vi "Prepare_ Trajectory.vi"(0 "reference in":refnum<class "Manipulator.lvclass">, 11 "error in (no error)":errorcluster) -> (4 "reference out":refnum<class "Manipulator.lvclass">, 6 "X":dbl[](array[numeric]), 8 "Y":dbl[](array[numeric]), 10 "Z":dbl[](array[numeric]), 15 "error out":errorcluster)   [LabVIEW 2014, in "Manipulator.lvclass"]
uses:
  Manipulator.lvclass
panel:
  out "c":dbl
  out "b":dbl
  out "a":dbl
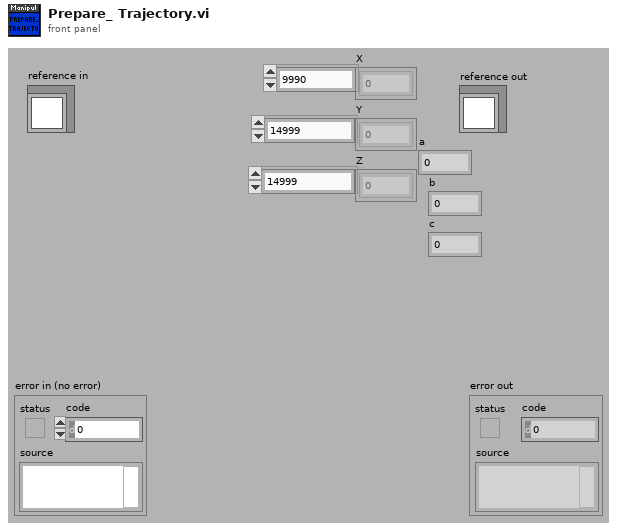
[diagram p1: front panel]
types:
  T1 = typedef "Manipulator.lvclass/ObjectAttributes.ctl" = cluster{"Coordinates":cluster{"X":dbl, "Y":dbl, "Z":dbl}, "Angles":cluster{"THETA_1":dbl, "THETA_2":dbl, "THETA_3":dbl, "THETA_4":dbl, "THETA_5":dbl, "THETA_6":dbl, "THETA_7":dbl, "THETA_8":dbl, "THETA_9":dbl, "THETA_10":dbl}, "Lengths":cluster{"a":dbl, "b":dbl, "c":dbl, "d":dbl, "e":dbl}, "Coordinates of joints":cluster{"A":cluster{"X":dbl, "Y":dbl, "Z":dbl}, "B":cluster{"X":dbl, "Y":dbl, "Z":dbl}, "C":cluster{"X":dbl, "Y":dbl, "Z":dbl}, "D":cluster{"X":dbl, "Y":dbl, "Z":dbl}}}
  T2 = cluster{"A":cluster{"X":dbl, "Y":dbl, "Z":dbl}, "B":cluster{"X":dbl, "Y":dbl, "Z":dbl}, "C":cluster{"X":dbl, "Y":dbl, "Z":dbl}, "D":cluster{"X":dbl, "Y":dbl, "Z":dbl}}
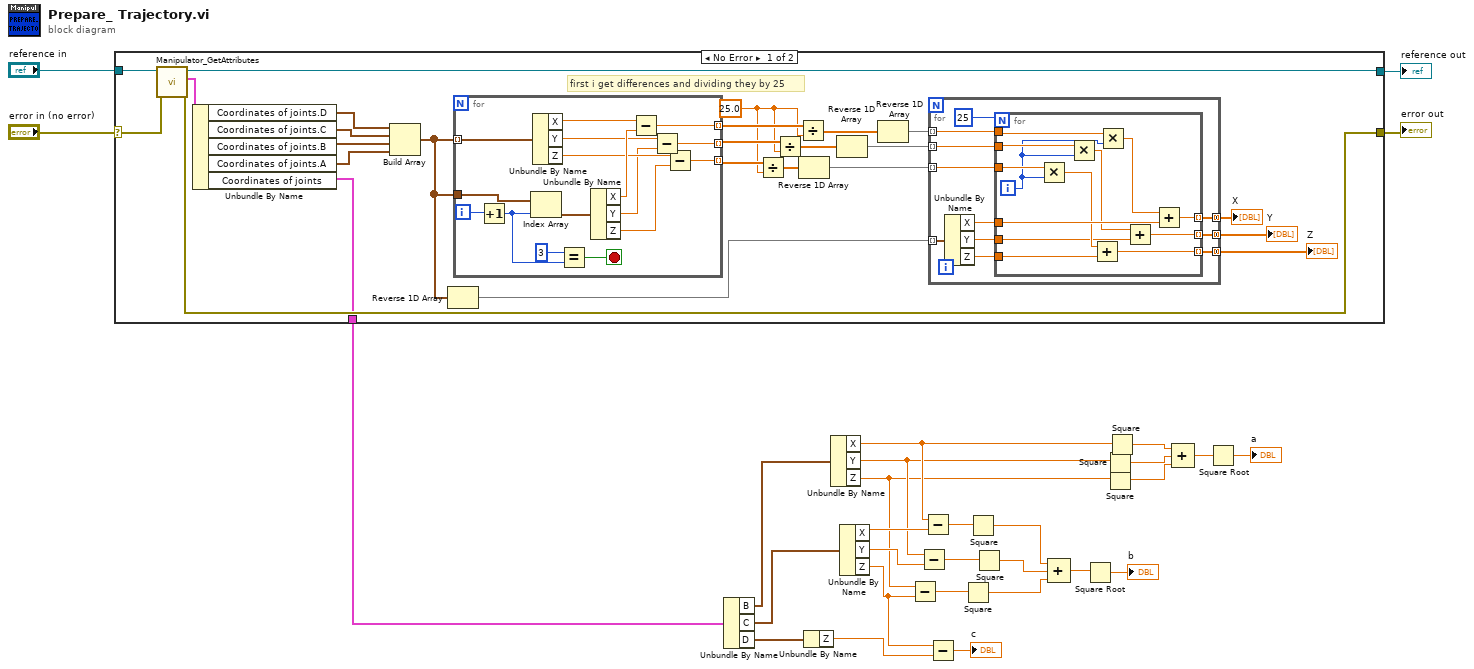
[diagram p0: block diagram]
diagram:
  n1 = case shown="No Error" "error in (no error)" {
    selector: "error in (no error)" -> [w53 w96]
    tunnel: [w31 w96] -> w28
    tunnel: [w52 w95] -> w26
    tunnel: "reference in" -> [w54 w95]
    tunnel: [w30 _] -> w1
    frame No Error {
      w43 = 25.0
      # "first i get differences and dividing they by 25"
      n2 = call "Manipulator_GetAttributes.vi"("error in (no error)"=w53, "reference in"=w54) -> ("error out"=w31:errorcluster, "Data"=w51:T1, "reference out"=w52:refnum<class "Manipulator.lvclass">)  [unwired: 6 in, 1 out]
      n3 = Unbundle By Name(w51) -> ("Coordinates of joints.D"=w47:cluster{"X":dbl, "Y":dbl, "Z":dbl}, "Coordinates of joints.C"=w48:cluster{"X":dbl, "Y":dbl, "Z":dbl}, "Coordinates of joints.B"=w49:cluster{"X":dbl, "Y":dbl, "Z":dbl}, "Coordinates of joints.A"=w50:cluster{"X":dbl, "Y":dbl, "Z":dbl}, "Coordinates of joints"=w30:T2)
      n4 = Build Array(w47, w48, w49, w50) -> (w39:cluster{"X":dbl, "Y":dbl, "Z":dbl}[])
      n5 = Reverse 1D Array(array=w39) -> (reversed array=w35:cluster{"X":dbl, "Y":dbl, "Z":dbl}[])
      n6 = for {
        tunnel: w39 -> [w94] mode=indexing
        tunnel: w39 -> [w91]
        tunnel: [w81] -> w46 mode=indexing
        tunnel: [w80] -> w45 mode=indexing
        tunnel: [w79] -> w44 mode=indexing
        i -> [w93]
        stop <- w89 stop-if-true
        n7 = Increment(x=w93) -> (x+1=w90:i32)
        n8 = Index Array(array=w91, index=w90) -> (element=w92:cluster{"X":dbl, "Y":dbl, "Z":dbl})
        n9 = Unbundle By Name(w94) -> ("X"=w87:dbl, "Y"=w85:dbl, "Z"=w84:dbl)
        n10 = Equal?(x=3, y=w90) -> (x = y?=w89:bool)
        n11 = Unbundle By Name(w92) -> ("X"=w86:dbl, "Y"=w82:dbl, "Z"=w83:dbl)
        n12 = Subtract(x=w87, y=w86) -> (x-y=w81:dbl)
        n13 = Subtract(x=w85, y=w82) -> (x-y=w80:dbl)
        n14 = Subtract(x=w84, y=w83) -> (x-y=w79:dbl)
      }
      n15 = Divide(x=w44, y=w43) -> (x/y=w40:dbl[])
      n16 = Divide(x=w45, y=w43) -> (x/y=w41:dbl[])
      n17 = Divide(x=w46, y=w43) -> (x/y=w42:dbl[])
      n18 = Reverse 1D Array(array=w40) -> (reversed array=w36:dbl[])
      n19 = Reverse 1D Array(array=w41) -> (reversed array=w37:dbl[])
      n20 = Reverse 1D Array(array=w42) -> (reversed array=w38:dbl[])
      n21 = for {
        tunnel: w38 -> [w65] mode=indexing
        tunnel: w37 -> [w64] mode=indexing
        tunnel: w36 -> [w63] mode=indexing
        tunnel: w35 -> [w62] mode=indexing
        tunnel: [w57] -> w34 mode=concatenating
        tunnel: [w56] -> w33 mode=concatenating
        tunnel: [w55] -> w32 mode=concatenating
        n22 = Unbundle By Name(w62) -> ("X"=w61:dbl, "Y"=w60:dbl, "Z"=w59:dbl)
        n23 = for {
          N: 25 -> [_]
          tunnel: w65 -> [w78]
          tunnel: w64 -> [w77]
          tunnel: w63 -> [w76]
          tunnel: w61 -> [w73]
          tunnel: w60 -> [w70]
          tunnel: w59 -> [w72]
          tunnel: [w68] -> w57 mode=indexing
          tunnel: [w67] -> w56 mode=indexing
          tunnel: [w66] -> w55 mode=indexing
          i -> [w75]
          n24 = Multiply(x=w76, y=w75) -> (x*y=w71:dbl)
          n25 = Multiply(x=w77, y=w75) -> (x*y=w69:dbl)
          n26 = Add(x=w71, y=w72) -> (x+y=w66:dbl)
          n27 = Multiply(x=w78, y=w75) -> (x*y=w74:dbl)
          n28 = Add(x=w69, y=w70) -> (x+y=w67:dbl)
          n29 = Add(x=w74, y=w73) -> (x+y=w68:dbl)
        }
      }
      "X" <- w34
      "Y" <- w33
      "Z" <- w32
    }
    frame Error {
    }
  }
  "error out" <- w28
  "reference out" <- w26
  n30 = Unbundle By Name(w1) -> ("B"=w25:cluster{"X":dbl, "Y":dbl, "Z":dbl}, "C"=w19:cluster{"X":dbl, "Y":dbl, "Z":dbl}, "D"=w5:cluster{"X":dbl, "Y":dbl, "Z":dbl})
  n31 = Unbundle By Name(w5) -> ("Z"=w3:dbl)
  n32 = Unbundle By Name(w25) -> ("X"=w18:dbl, "Y"=w14:dbl, "Z"=w11:dbl)
  n33 = Unbundle By Name(w19) -> ("X"=w17:dbl, "Y"=w13:dbl, "Z"=w4:dbl)
  n34 = Subtract(x=w11, y=w4) -> (x-y=w12:dbl)
  n35 = Subtract(x=w14, y=w13) -> (x-y=w15:dbl)
  n36 = Subtract(x=w18, y=w17) -> (x-y=w16:dbl)
  n37 = Subtract(x=w4, y=w3) -> (x-y=→"c":dbl)
  n38 = Square(x=w12) -> (x^2=w8:dbl)
  n39 = Square(x=w16) -> (x^2=w10:dbl)
  n40 = Square(x=w15) -> (x^2=w9:dbl)
  n41 = Compound Arithmetic op=ADD(w10, w9, w8) -> (w7:dbl)
  n42 = Square Root(x=w7) -> (sqrt(x)=→"b":dbl)
  n43 = Square(x=w14) -> (x^2=w23:dbl)
  n44 = Square(x=w11) -> (x^2=w22:dbl)
  n45 = Square(x=w18) -> (x^2=w24:dbl)
  n46 = Compound Arithmetic op=ADD(w24, w23, w22) -> (w21:dbl)
  n47 = Square Root(x=w21) -> (sqrt(x)=→"a":dbl)
